vi "iotest.vi"   [LabVIEW 2014]
types:
  T1 = enum16{"big-endian, network order", "native, host order", "little-endian"}
  T2 = enum16{"open", "replace", "create", "open or create", "replace or create", "replace or create with confirmation"}
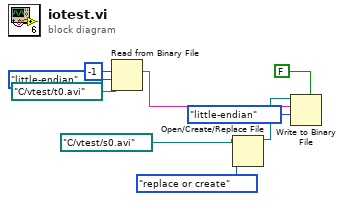
[diagram p0: block diagram]
diagram:
  n1 = Read from Binary File(9:T1."little-endian" ("byte order (0:big-endian, network order)"), 10:-1 ("count (1)"), 11:path "C:/vtest/t0.avi" ("file (use dialog)")) -> (2:w5:string)  [unwired: 3 in, 3 out]
  n2 = Open/Create/Replace File(file path (use dialog)=path "C:/vtest/s0.avi" ("file (use dialog)"), operation (0:open)=T2."replace or create") -> (refnum out=w9:refnum<file>)  [unwired: 4 in, 2 out]
  n3 = Write to Binary File(file (use dialog)=w9, data=w5, 5:FALSE ("prepend array or string size? (T)"), 9:T1."little-endian" ("byte order (0:big-endian, network order)")) -> ()  [unwired: 2 in, 3 out]
